vi "TP FPGA.vi"   [LabVIEW 2018]
uses:
  <vilib>/rvi/Emulation/niFpgaGetClockAttributes.vi
  <vilib>/rvi/Emulation/niFpgaSctlEmulationGetInTimedLoop.vi
  <vilib>/rvi/Emulation/niFpgaEmulationReportErrorSimple.vi
  <vilib>/rvi/eio/common/nirviEmuTemplateMethod_errors.vi
  <vilib>/rvi/Emulation/niFpgaCriticalErrorInLSC.vi
  <vilib>/eio/EIONode/EIONode.xnode
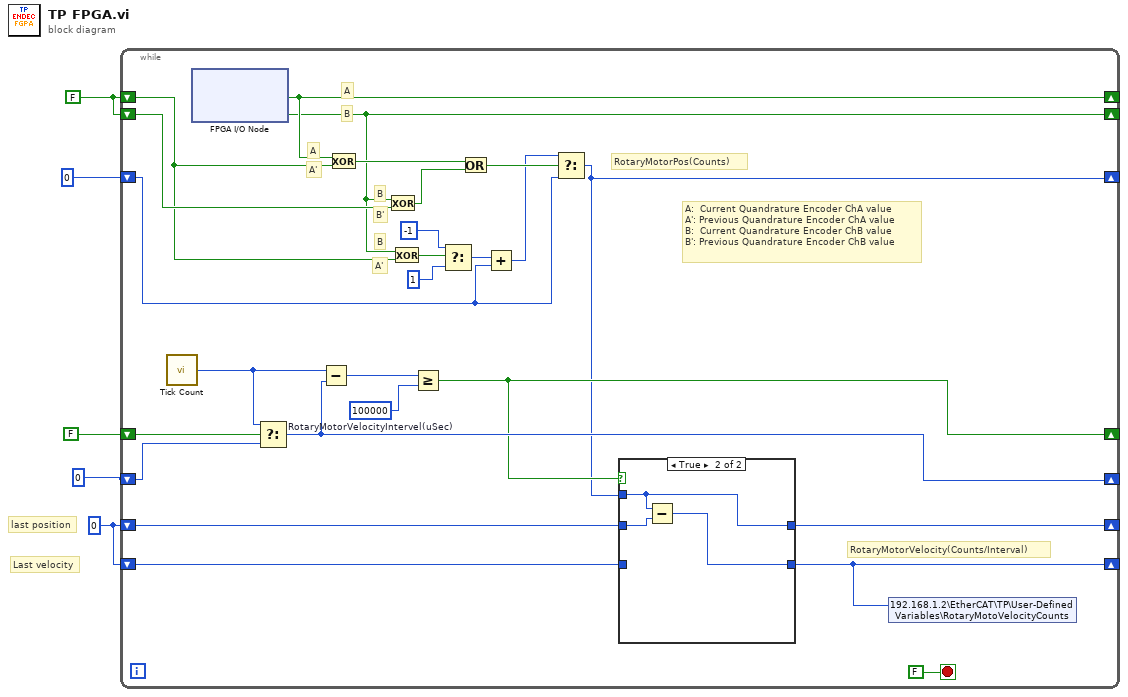
[diagram p0: block diagram]
diagram:
  w1 = i16 0 ("s? t:f")
  w5 = FALSE
  # "Last velocity"
  # "last position"
  n1 = while {
    shift-right: [w26] -> _
    shift-left: w5 -> [w29]
    shift-right: [w30] -> _
    shift-left: w5 -> [w25]
    shift-right: [w10] -> _
    shift-left: i16 0 -> [w20]
    shift-right: [w11] -> _
    shift-left: FALSE -> [w17]
    shift-right: [w12] -> _
    shift-left: u32 0 ("f") -> [w16]
    shift-right: [w9] -> _
    shift-left: w1 -> [w8]
    shift-right: [w6] -> _
    shift-left: w1 -> [w7]
    stop <- FALSE stop-if-true
    w13 = u32 100000  # RotaryMotorVelocityIntervel(uSec)
    # "RotaryMotorVelocity(Counts/Interval)"
    # "RotaryMotorPos(Counts)"
    # "A:  Current Quandrature Encoder ChA value\nA': Previous Quandrature Encoder ChA value\nB:  Current Quandrature Encoder ChB value\nB': Previous Quandrature Encoder ChB value"
    # "A'"
    # "B"
    # "B'"
    # "B"
    # "A'"
    # "A"
    # "B"
    # "A"
    n2 = call "Tick Count"() -> ("Tick Count(Ticks)"=w15:u32)
    n3 = xnode "FPGA I/O Node"() -> ("Mod5/DI0"=w30:bool, "Mod5/DI1"=w26:bool)  [unwired: 2 in, 2 out]
    n4 = Select(t=w15, s=w17, f=w16) -> (s? t:f=w12:u32)
    n5 = Subtract(x=w15, y=w12) -> (x-y=w14:u32)
    n6 = Exclusive Or(1:w25, 2:w30) -> (0:w28:bool)
    n7 = Exclusive Or(1:w29, 2:w26) -> (0:w27:bool)
    n8 = Exclusive Or(1:w25, 2:w26) -> (0:w24:bool)
    n9 = Greater Or Equal?(x=w14, y=w13) -> (x >= y?=w11:bool)
    n10 = Select(t=i16 -1, s=w24, f=i16 1) -> (s? t:f=w21:i16)
    n11 = Or(x=w28, y=w27) -> (x .or. y?=w19:bool)
    n12 = Add(x=w21, y=w20) -> (x+y=w18:i16)
    n13 = Select(t=w18, s=w19, f=w20) -> (s? t:f=w10:i16)
    n14 = case shown="True" w11 {
      tunnel: w10 -> [_ w36]
      tunnel: [w33 w36] -> w9
      tunnel: w8 -> [w33 w35]
      tunnel: w7 -> [w32 _]
      tunnel: [w32 w34] -> w6
      frame False {
      }
      frame True {
        n15 = Subtract(x=w36, y=w35) -> (x-y=w34:i16)
      }
    }
    n16 = shared-variable "192.168.1.2\\EtherCAT\\TP\\User-Defined Variables\\RotaryMotoVelocityCounts"(w6) -> ()  [unwired: 1 in, 1 out]
  }
